vi "Check and Override Channel Configuration.vi"(8 "error in (no error)":errorcluster, 10 "Custom Config Data in":u8[](array[numeric]) format="%.0x", 11 "CIF_NIChn_FifoCAN in":refnum<class "CIF_NIChn_FifoCAN.lvclass">) -> (0 "error out":errorcluster, 2 "Custom Config Data out":u8[](array[numeric]) format="%.0x", 3 "CIF_NIChn_FifoCAN out":refnum<class "CIF_NIChn_FifoCAN.lvclass">)   [LabVIEW 2021, in "CIF_NIChn_FifoCAN.lvclass"]
uses:
  CIF_NIChn_FifoCAN.lvclass
  <vilib>/CIF Foundation/CIF Utilities/DataTypes/Unflatten U64.vi
  <vilib>/CIF Foundation/CIF Utilities/DataTypes/Flatten U64.vi
  CIF_NIChn_FifoCAN.lvclass/CIF_NIChn_FifoCAN.ctl
  ChannelCommon/ChannelCommon.lvlib
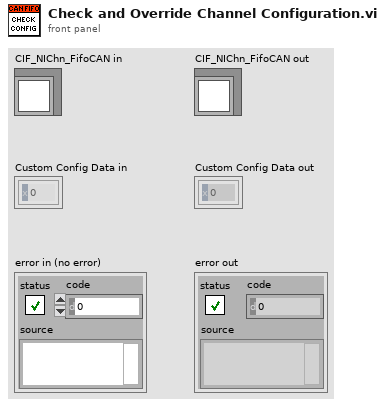
[diagram p1: front panel]
types:
  T1 = typedef "ChannelCommon.lvlib/FIFO Config.ctl" = cluster{"Max Bytes/Msg":u64, "Max Msg/FIFO":u64, "Flags":u64}
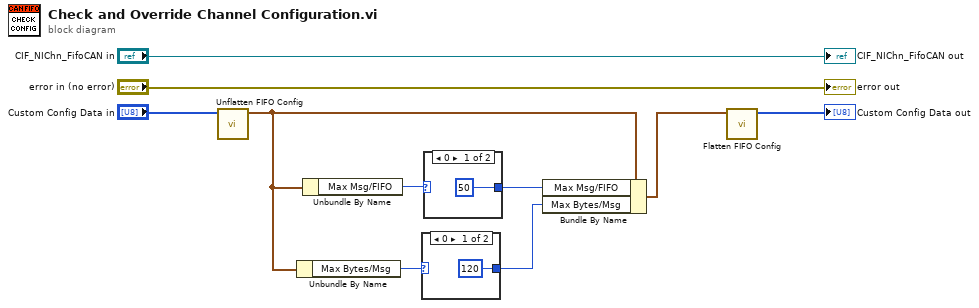
[diagram p0: block diagram]
diagram:
  n1 = call "Unflatten FIFO Config.vi"("Flattened Data in"="Custom Config Data in") -> ("FIFO Config out"=w6:T1)  [unwired: 9 in, 1 out]
  n2 = Unbundle By Name(w6) -> ("Max Bytes/Msg"=w8:u64)
  n3 = Unbundle By Name(w6) -> ("Max Msg/FIFO"=w7:u64)
  n4 = case shown="0" w8 {
    selector: w8 -> [_ w12]
    tunnel: [u64 120 ("y") w12] -> w3
    frame 0 {
    }
    frame 1, Default {
    }
  }
  n5 = case shown="0" w7 {
    selector: w7 -> [_ w14]
    tunnel: [u64 50 ("y") w14] -> w4
    frame 0 {
    }
    frame 1, Default {
    }
  }
  n6 = Bundle By Name(cluster=w6, "Max Msg/FIFO"=w4, "Max Bytes/Msg"=w3) -> (w5:T1)
  n7 = call "Flatten FIFO Config.vi"("FIFO Config in"=w5) -> ("Flattened FIFO Config"=→"Custom Config Data out":u8[])  [unwired: 10 in]
  "error out" <- "error in (no error)"
  "CIF_NIChn_FifoCAN out" <- "CIF_NIChn_FifoCAN in"
